vi "Dynamic Class Loading.vi"() -> ()   [LabVIEW 2015]
uses:
  Square/Square.lvclass
  Square/Square.lvclass/Square.ctl
  Square/Read Name.vi
panel:
  in  "class path":path=path "C:/GIT/SquareBattle/Builds/Squares/Expand.lvclass"
  out "error out 2":errorcluster
  out "Name":string
  out "error out":errorcluster
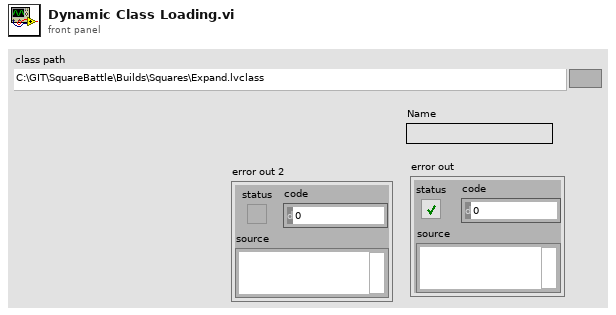
[diagram p1: front panel]
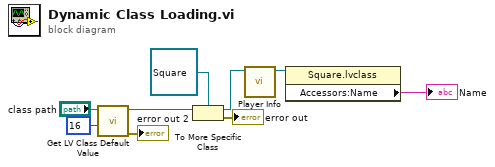
[diagram p0: block diagram]
diagram:
  n1 = call <vilib>:"Get LV Class Default Value.vi"("options"=u32 16, "class path"="class path") -> ("error out"=→"error out 2":errorcluster, "object"=w9:refnum<class>)  [unwired: 8 in]
  n2 = To More Specific Class(target class=refnum<class "Square.lvclass"> refnum ("Square.lvclass"), reference=w9) -> (specific class reference=w5:refnum<class "Square.lvclass">, error out=→"error out":errorcluster)  [unwired: 1 in]
  n3 = call-dynamic "Player Info.vi"("Square in"=w5) -> ("Square out"=w4:refnum<class "Square.lvclass">)  [unwired: 10 in]
  n4 = property class="Square.lvclass"(reference=w4) -> ("Accessors:Name"=→"Name":string)  [unwired: 1 in, 2 out]
